vi "SeCrTs-RD File & Folder.vi"(8 "error in (no error)":errorcluster) -> (0 "error out":errorcluster, 3 "File Output":T1)   [LabVIEW 2022 SP3]
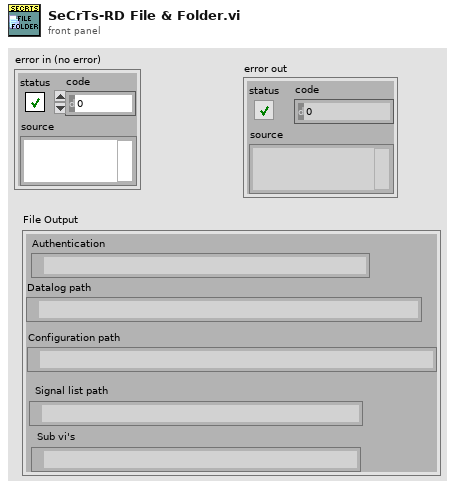
[diagram p1: front panel]
types:
  T1 = cluster{"Datalog path":path, "Configuration path":path, "Signal list path":path, "Sub vi's":path, "Authentication":path}
  T2 = enum32{"invalid app kind", "Development System", "Run Time System", "Student Edition", "Embedded LabVIEW", "Evaluation", "Custom"}
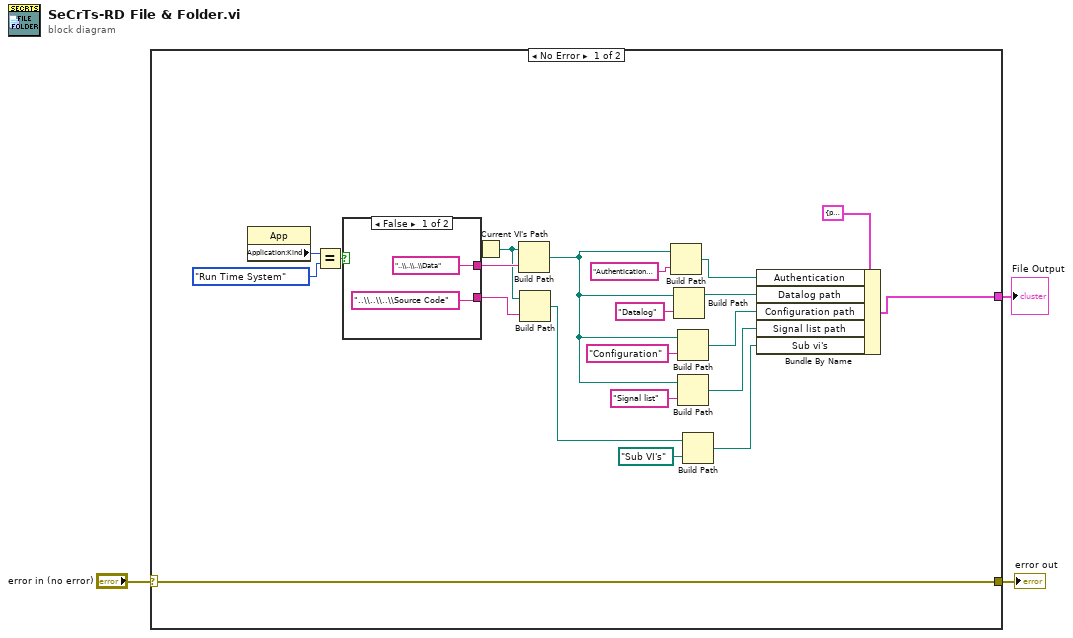
[diagram p0: block diagram]
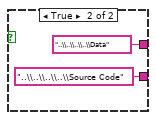
[diagram p2: hidden frame]
diagram:
  n1 = case shown="No Error" "error in (no error)" {
    selector: "error in (no error)" -> [w17 _]
    tunnel: [w17 _] -> w2
    tunnel: [w16 _] -> w1
    frame No Error {
      n2 = property class="App"() -> ("Application:Kind"=w23:T2)  [unwired: 2 in, 2 out]
      n3 = Equal?(x=w23, y=T2."Run Time System") -> (x = y?=w21:bool)
      n4 = case shown="False" w21 {
        tunnel: ["..\\..\\..\\Data" ("name or relative path") "..\\..\\..\\..\\Data" ("name or relative path")] -> w24
        tunnel: ["..\\..\\..\\Source Code" ("name or relative path") "..\\..\\..\\..\\Source Code" ("name or relative path")] -> w11
        frame False {
        }
        frame True {
        }
      }
      n5 = Current VI's Path() -> (path=w10:path)
      n6 = Build Path(base path=w10, name or relative path=w24) -> (appended path=w6:path)
      n7 = Build Path(base path=w10, name or relative path=w11) -> (appended path=w9:path)
      n8 = Build Path(base path=w6, name or relative path="Authentication Details") -> (appended path=w4:path)
      n9 = Build Path(base path=w6, name or relative path="Datalog") -> (appended path=w18:path)
      n10 = Build Path(base path=w6, name or relative path="Configuration") -> (appended path=w13:path)
      n11 = Build Path(base path=w6, name or relative path="Signal list") -> (appended path=w12:path)
      n12 = Build Path(base path=w9, name or relative path=path "Sub VI's") -> (appended path=w7:path)
      n13 = Bundle By Name(cluster=T1 {"Datalog path"=path "", "Configuration path"=path "", "Signal list path"=path "", "Sub vi's"=path "", "Authentication"=path ""} ("Cluster"), "Authentication"=w4, "Datalog path"=w18, "Configuration path"=w13, "Signal list path"=w12, "Sub vi's"=w7) -> (w16:T1)
    }
    frame Error {
    }
  }
  "error out" <- w2
  "File Output" <- w1
